vi "getSubArray1D.vi"(8 "error in (no error)":errorcluster, 9 "Index Array Cluster":cluster{"Idx of Dim 0":i32[]}, 11 "1D Array":dbl[](array[numeric])) -> (0 "error out":errorcluster, 3 "Sub-Array":dbl[](array[numeric]))   [LabVIEW 2016]
doc: "Get the sub-array of the specific 1D array based on the index array."
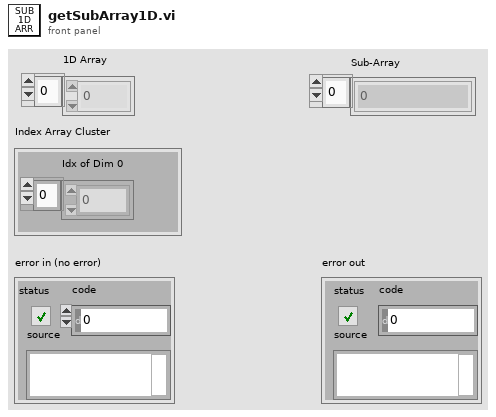
[diagram p1: front panel]
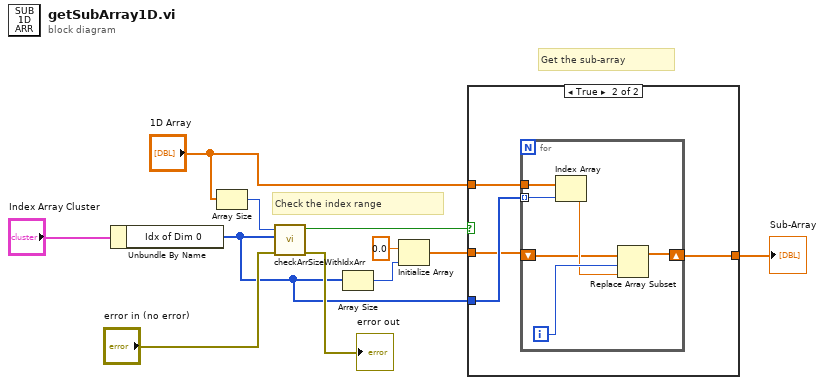
[diagram p0: block diagram]
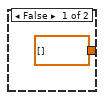
[diagram p2: hidden frame]
diagram:
  # "Get the sub-array"
  # "Check the index range"
  n1 = Unbundle By Name("Index Array Cluster") -> ("Idx of Dim 0"=w5:i32[])
  n2 = Array Size(array="1D Array") -> (size(s)=w1:i32)
  n3 = call "checkArrSizeWithIdxArr.vi"("error in (no error)"="error in (no error)", "Idx Array"=w5, "Array Size"=w1) -> ("error out"=→"error out":errorcluster, "In Spec"=w9:bool)  [unwired: 7 in]
  n4 = Array Size(array=w5) -> (size(s)=w6:i32)
  n5 = Initialize Array(0.0 ("element"), w6) -> (w4:dbl[])
  n6 = case shown="True" w9 {
    tunnel: "1D Array" -> [_ w16]
    tunnel: w5 -> [_ w15]
    tunnel: w4 -> [_ w14]
    tunnel: [dbl[] [] w13] -> w3
    frame False {
    }
    frame True {
      n7 = for {
        tunnel: w16 -> [w22]
        tunnel: w15 -> [w21] mode=indexing
        shift-right: [w17] -> w13
        shift-left: w14 -> [w18]
        i -> [w20]
        n8 = Index Array(array=w22, index=w21) -> (element=w19:dbl)
        n9 = Replace Array Subset(array=w18, new element=w19, index=w20) -> (w17:dbl[])
      }
    }
  }
  "Sub-Array" <- w3
